vi "Lab Arreglos-3.vi"() -> ()   [LabVIEW 2018]
panel:
  in  "stop":bool
  out "Array":sgl[](array[numeric])
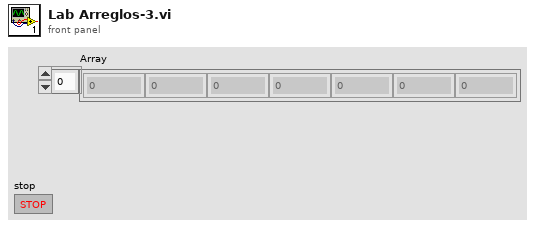
[diagram p1: front panel]
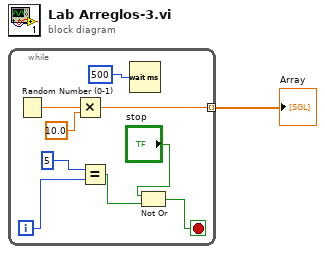
[diagram p0: block diagram]
diagram:
  n1 = while {
    tunnel: [w8] -> w1 mode=indexing
    i -> [w10]
    stop <- w4 stop-if-true
    n2 = Random Number (0-1)() -> (number: 0 to 1=w6:dbl)
    n3 = Multiply(x=w6, y=10.0) -> (x*y=w8:dbl)
    n4 = Equal?(x=5, y=w10) -> (x = y?=w5:bool)
    n5 = Wait (ms)(milliseconds to wait=u32 500) -> ()  [unwired: 1 out]
    n6 = Not Or(1:w5, 2:"stop") -> (0:w4:bool)
  }
  "Array" <- w1
